vi "Read Temperature C.vi"(7 "Use Cached Data?":bool, 8 "Error In":errorcluster, 10 "Device Name":string, 11 "Nest Config":T1) -> (0 "Error Out":errorcluster, 2 "Current Temp (C)":dbl, 3 "Nest Config":T1)   [LabVIEW 2013, in "LVH-Nest.lvlib"]
doc: "Read temperature from specified Nest device."
uses:
  LVH-Nest.lvlib
  Private/Type Defs/Nest Config.ctl
  <vilib>/httpClient/ClientHandle.ctl
  Private/Type Defs/Session Data.ctl
  <vilib>/httpClient/LabVIEWHTTPClient.lvlib
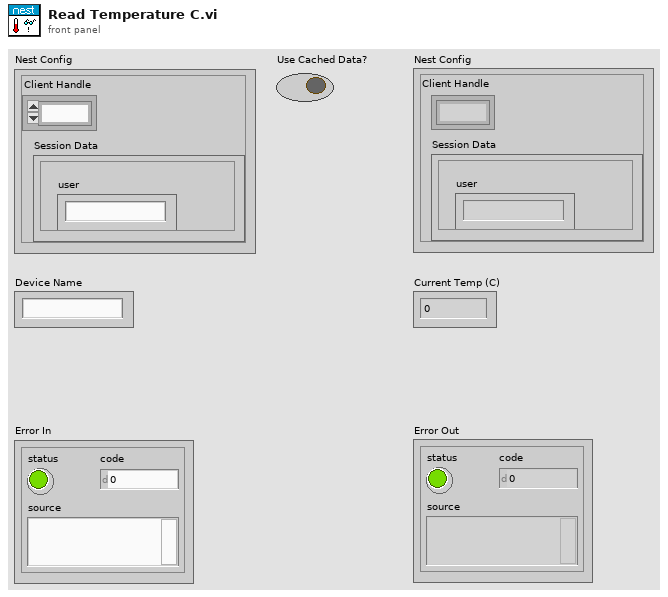
[diagram p1: front panel]
types:
  T1 = typedef "LVH-Nest.lvlib/Nest Config.ctl" = cluster{"Client Handle":T2, "Session Data":T3}
  T2 = typedef "LabVIEWHTTPClient.lvlib/ClientHandle.ctl" = refnum<k1>
  T3 = typedef "LVH-Nest.lvlib/Session Data.ctl" = cluster{"is_superuser":bool, "is_staff":bool, "urls":cluster{"transport_url":string, "rubyapi_url":string, "weather_url":string, "log_upload_url":string, "support_url":string}, "limits":cluster{"thermostats_per_structure":u32, "structures":u32, "thermostats":u32, "smoke_detectors":u32, "smoke_detectors_per_structure":u32}, "access_token":string, "userid":string, "expires_in":string, "email":string, "user":string, "language":string}
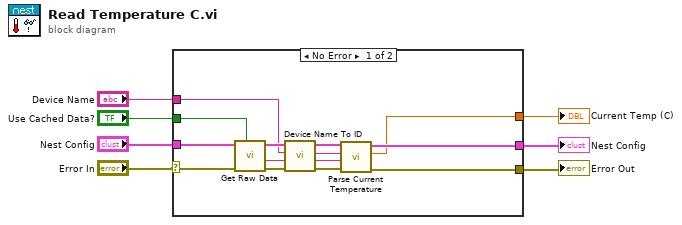
[diagram p0: block diagram]
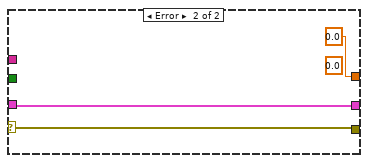
[diagram p2: hidden frame]
diagram:
  n1 = case shown="No Error" "Error In" {
    selector: "Error In" -> [w8 w24]
    tunnel: "Use Cached Data?" -> [w21 _]
    tunnel: "Nest Config" -> [w20 w23]
    tunnel: "Device Name" -> [w18 _]
    tunnel: [w11 w24] -> w4
    tunnel: [w10 w23] -> w3
    tunnel: [w9 0.0 ("Current Temp")] -> w2
    frame No Error {
      n2 = call "Get Raw Data.vi"("Use Cached Data?"=w21, "Error In"=w8, "Nest Config"=w20) -> ("Error Out"=w17:errorcluster, "Data"=w16:string, "Nest Config"=w19:T1)  [unwired: 6 in]
      n3 = call "Device Name To ID.vi"("Error In"=w17, "Data"=w16, "Device Name"=w18, "Nest Config"=w19) -> ("Error Out"=w14:errorcluster, "Data"=w13:string, "Device ID"=w12:string, "Nest Config"=w15:T1)  [unwired: 4 in]
      n4 = call "Parse Current Temperature.vi"("Error In"=w14, "Data"=w13, "Device ID"=w12, "Nest Config"=w15) -> ("Error Out"=w11:errorcluster, "Current Temp"=w9:dbl, "Nest Config"=w10:T1)  [unwired: 4 in, 1 out]
    }
    frame Error {
      (unwired) 0.0
    }
  }
  "Error Out" <- w4
  "Nest Config" <- w3
  "Current Temp (C)" <- w2
